vi "MissingInProject.vi"(8 "error in":errorcluster, 11 "File Path":path) -> (0 "error out":errorcluster, 1 "Missing Files":string, 2 "Passed":bool, 3 "Debug":string)   [LabVIEW 2020, in "Missing in Project Tests.lvlib"]
uses:
  Missing in Project Tests.lvlib
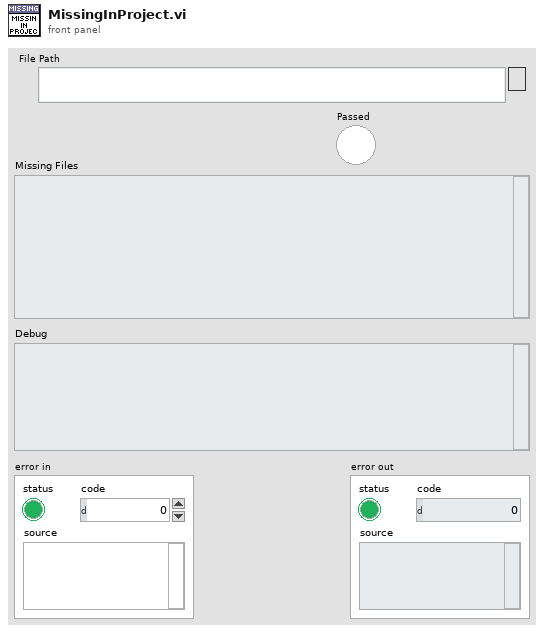
[diagram p1: front panel]
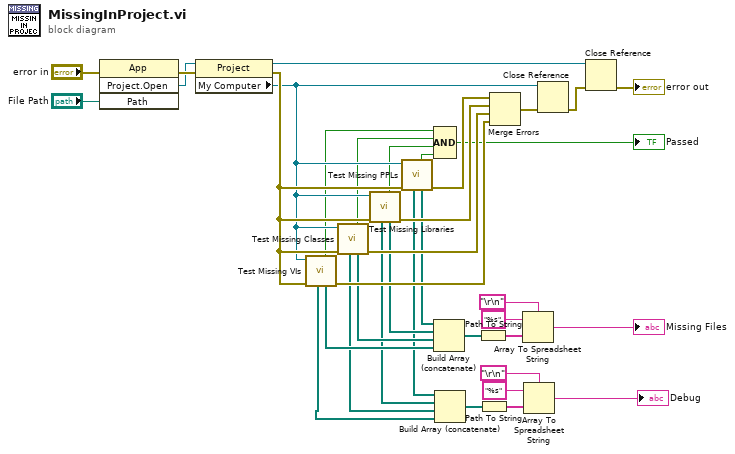
[diagram p0: block diagram]
diagram:
  n1 = invoke class="App" method="Project.Open"(error in="error in", "Path"="File Path") -> (error out=w37:errorcluster, "Project:Open"=w28:refnum<vi>)  [unwired: 2 in, 2 out]
  n2 = property class="Project"(reference=w28, error in=w37) -> (reference out=w26:refnum<vi>, error out=w29:errorcluster, "My Computer"=w25:refnum<vi>)
  n3 = call "Test Missing VIs.vi"("error in"=w29, "My Computer"=w25) -> ("error out"=w32:errorcluster, "Missing items"=w16:path[], "Pass"=w20:bool, "Debug"=w4:path[])  [unwired: 6 in]
  n4 = call "Test Missing Classes.vi"("error in"=w29, "My Computer"=w25) -> ("error out"=w33:errorcluster, "Missing items from LabVIEW project"=w17:path[], "Pass"=w21:bool, "Debug"=w3:path[])  [unwired: 6 in]
  n5 = call "Test Missing Libraries.vi"("error in"=w29, "My Computer"=w25) -> ("error out"=w34:errorcluster, "Missing items from LabVIEW project"=w18:path[], "Pass"=w22:bool, "Debug"=w2:path[])  [unwired: 6 in]
  n6 = call "Test Missing PPLs.vi"("error in"=w29, "My Computer"=w25) -> ("error out"=w35:errorcluster, "Missing items from LabVIEW project"=w19:path[], "Pass"=w23:bool, "Debug"=w1:path[])  [unwired: 6 in]
  n7 = Compound Arithmetic op=AND(w20, w21, w22, w23) -> (→"Passed":bool)
  n8 = Build Array (concatenate)(w19, w18, w17, w16) -> (w15:path[])
  n9 = Build Array (concatenate)(w1, w2, w3, w4) -> (w6:path[])
  n10 = Path To String(path=w15) -> (string=w14:string[])
  n11 = Path To String(path=w6) -> (string=w7:string[])
  n12 = Merge Errors(w35, w34, w33, w32) -> (w31:errorcluster)
  n13 = Array To Spreadsheet String(delimiter (Tab)="\r\n", array=w14, 3:"%s" ("format string")) -> (spreadsheet string=→"Missing Files":string)
  n14 = Array To Spreadsheet String(delimiter (Tab)="\r\n", array=w7, 3:"%s" ("format string")) -> (spreadsheet string=→"Debug":string)
  n15 = Close Reference(reference=w25, error in (no error)=w31) -> (error out=w36:errorcluster)
  n16 = Close Reference(reference=w26, error in (no error)=w36) -> (error out=→"error out":errorcluster)
